vi "RegisterForMessage.vi"(8 "error in (no error)":errorcluster, 9 "message names":string[](array[string]), 10 "process name":string, 11 "Qbus in":refnum<class "Qbus.lvclass">) -> (0 "error in (no error)":errorcluster, 3 "Qbus out":refnum<class "Qbus.lvclass">)   [LabVIEW 2017, in "Qbus.lvclass"]
doc: "Subscribes a process to receive one or more types of messages in its message queue whenever another process broadcasts those messages."
uses:
  <vilib>/addons/Qbus/Qbus.lvclass
  <vilib>/addons/Qbus/Qbus.lvclass/Qbus.ctl
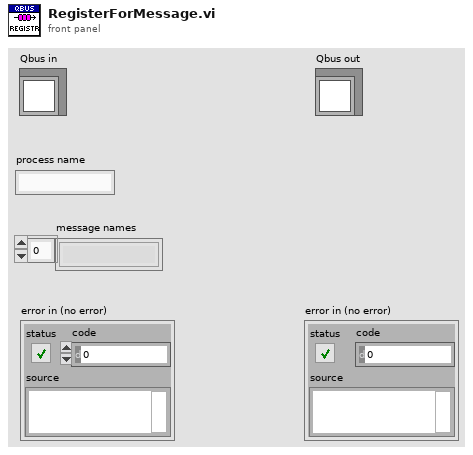
[diagram p1: front panel]
types:
  T1 = typedef "Qbus.lvclass/data.ctl" = cluster{"Queues":variant, "Subscriptions":variant, "MasterQ":string}
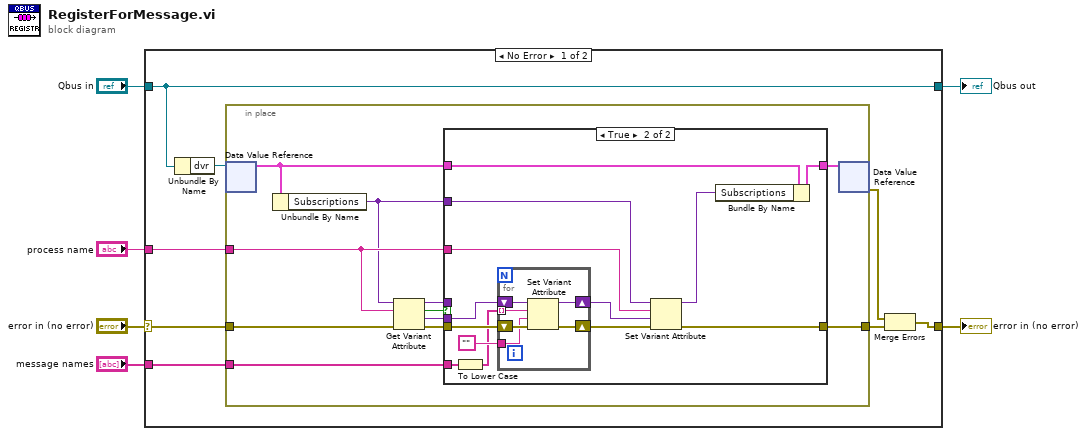
[diagram p0: block diagram]
diagram:
  n1 = case shown="No Error" "error in (no error)" {
    selector: "error in (no error)" -> [w10 w48]
    tunnel: [w9 w48] -> w5
    tunnel: [w14 w47] -> w3
    tunnel: "Qbus in" -> [w14 w47]
    tunnel: "process name" -> [w12 _]
    tunnel: "message names" -> [w7 _]
    frame No Error {
      n2 = Unbundle By Name(w14) -> ("dvr"=w13:refnum<data-value>)
      n3 = in-place {
        in-place-border: w10 -> [w25]
        in-place-border: w12 -> [w19]
        in-place-border: [w18] -> w8
        in-place-border: w7 -> [w15]
        n4 = in-place-dvr #1(w13) -> (w21:T1)  [unwired: 1 out]
        n5 = Unbundle By Name(w21) -> ("Subscriptions"=w17:variant)
        n6 = Get Variant Attribute(Variant=w17, name=w19, error in=w25) -> (duplicate Variant=w20:variant, found=w24:bool, value=w16:variant, error out=w23:errorcluster)  [unwired: 1 in]
        n7 = case shown="True" w24 {
          tunnel: w23 -> [w27 w40]
          tunnel: [w26 w37] -> w22
          tunnel: w21 -> [w26 w38]
          tunnel: w20 -> [_ _]
          tunnel: w17 -> [_ w33]
          tunnel: w19 -> [_ w30]
          tunnel: [w27 w31] -> w18
          tunnel: w16 -> [_ w39]
          tunnel: w15 -> [_ w36]
          frame False {
          }
          frame True {
            n8 = To Lower Case(string=w36) -> (all lower case string=w34:string[])
            n9 = for {
              shift-right: [w44] -> w29
              shift-left: w40 -> [w46]
              shift-right: [w43] -> w28
              shift-left: w39 -> [w45]
              tunnel: w34 -> [w42] mode=indexing
              tunnel: "" -> [w41]
              n10 = Set Variant Attribute(Variant=w45, name=w42, value=w41, error in=w46) -> (Variant out=w43:variant, error out=w44:errorcluster)  [unwired: 1 out]
            }
            n11 = Set Variant Attribute(Variant=w33, name=w30, value=w28, error in=w29) -> (Variant out=w32:variant, error out=w31:errorcluster)  [unwired: 1 out]
            n12 = Bundle By Name(cluster=w38, "Subscriptions"=w32) -> (w37:T1)
          }
        }
        n13 = in-place-dvr #1(w22) -> (w11:errorcluster)  [unwired: 1 out]
      }
      n14 = Merge Errors(w11, w8) -> (w9:errorcluster)
    }
    frame Error {
    }
  }
  "error in (no error)" <- w5
  "Qbus out" <- w3
